vi "_testFileFlash.vi"(8 "speed":u32=4000, 9 "Path":path, 11 "implement":enum16{"Burning", "Erase"}(ring)) -> (10 "cmdStr out":string)   [LabVIEW 2020, in "LvJLinkARM.lvlib"]
uses:
  LvJLinkARM.lvlib
panel:
  out "return 5":i32
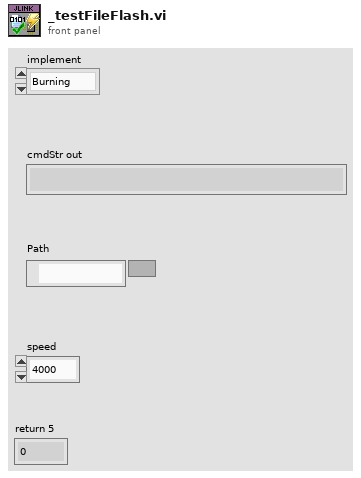
[diagram p1: front panel]
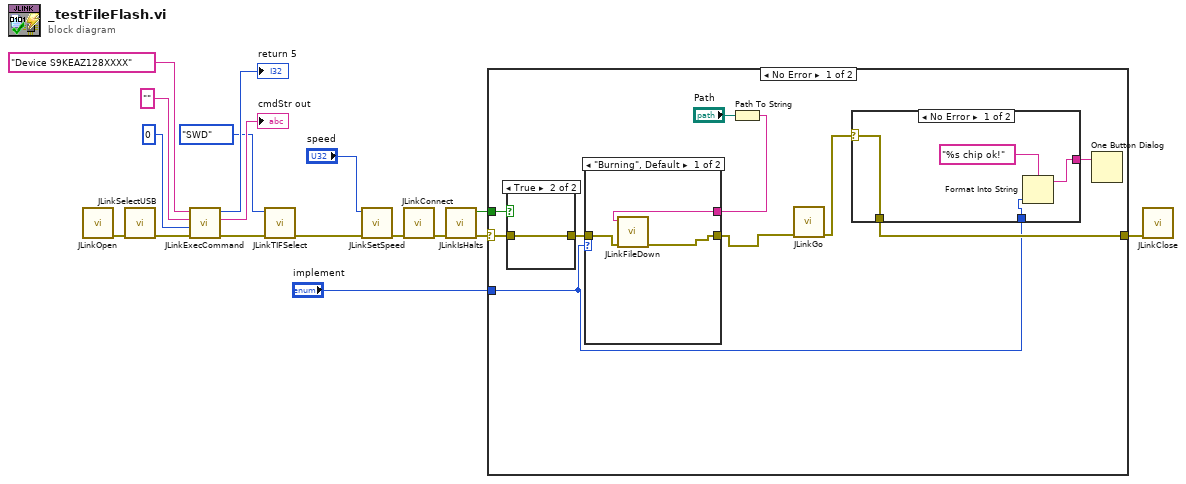
[diagram p0: block diagram]
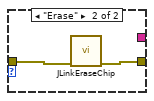
[diagram p2: hidden frame]
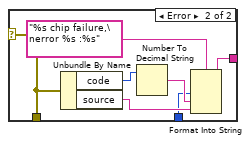
[diagram p3: hidden frame]
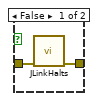
[diagram p4: hidden frame]
diagram:
  n1 = call "JLinkOpen.vi"() -> ("error out"=w7:errorcluster)  [unwired: 11 in]
  n2 = call "JLinkSelectUSB.vi"("error in (no error)"=w7) -> ("error out"=w8:errorcluster)  [unwired: 10 in]
  n3 = call "JLinkExecCommand.vi"("error in (no error)"=w8, "BufferSize"=0, "sError"="", "cmdStr"="Device S9KEAZ128XXXX") -> ("error out"=w11:errorcluster, "cmdStr out"=→"cmdStr out":string, "return"=→"return 5":i32)  [unwired: 5 in]
  n4 = call "JLinkTIFSelect.vi"("error in (no error)"=w11, "interface"=enum16{"JTAG", "SWD"}."SWD") -> ("error out"=w9:errorcluster)  [unwired: 9 in]
  n5 = call "JLinkSetSpeed.vi"("error in (no error)"=w9, "speed"="speed") -> ("error out"=w10:errorcluster)  [unwired: 9 in]
  n6 = call "JLinkConnect.vi"("error in (no error)"=w10) -> ("error out"=w5:errorcluster)  [unwired: 10 in]
  n7 = call "JLinkIsHalts.vi"("error in (no error)"=w5) -> ("error out"=w4:errorcluster, "inHalts？"=w3:bool)  [unwired: 9 in]
  n8 = case shown="No Error" w4 {
    selector: w4 -> [w26 w47]
    tunnel: w3 -> [w27 _]
    tunnel: [w23 w47] -> w2
    tunnel: "implement" -> [w18 _]
    frame No Error {
      n9 = case shown="True" w27 {
        tunnel: w26 -> [w45 w46]
        tunnel: [w44 w46] -> w25
        frame False {
          n10 = call "JLinkHalts.vi"("error in (no error)"=w45) -> ("error out"=w44:errorcluster)  [unwired: 9 in, 1 out]
        }
        frame True {
        }
      }
      n11 = Path To String(path="Path") -> (string=w21:string)
      n12 = case shown="\"Burning\", Default" w18 {
        tunnel: w25 -> [w29 w32]
        tunnel: [w28 w31] -> w20
        tunnel: w21 -> [w30 _]
        frame "Burning", Default {
          n13 = call "JLinkFileDown.vi"("error in (no error)"=w29, "sFileName"=w30) -> ("error out"=w28:errorcluster)  [unwired: 9 in]
        }
        frame "Erase" {
          n14 = call "JLinkEraseChip.vi"("error in (no error)"=w32) -> ("error out"=w31:errorcluster)  [unwired: 10 in]
        }
      }
      n15 = call "JLinkGo.vi"("error in (no error)"=w20) -> ("error out"=w19:errorcluster)  [unwired: 10 in]
      n16 = case shown="No Error" w19 {
        selector: w19 -> [w36 w43]
        tunnel: [w36 w43] -> w23
        tunnel: [w33 w42] -> w22
        tunnel: w18 -> [w35 w37]
        frame No Error {
          n17 = Format Into String(format string="%s chip ok!" ("message"), w35) -> (resulting string=w33:string)  [unwired: 2 in, 1 out]
        }
        frame Error {
          n18 = Unbundle By Name(w43) -> ("code"=w40:i32, "source"=w38:string)
          n19 = Number To Decimal String(number=w40) -> (decimal integer string=w39:string)  [unwired: 1 in]
          n20 = Format Into String(format string="%s chip failure,\nerror %s :%s", w37, w39, w38) -> (resulting string=w42:string)  [unwired: 2 in, 1 out]
        }
      }
      n21 = One Button Dialog(message=w22) -> ()  [unwired: 1 in, 1 out]
    }
    frame Error {
    }
  }
  n22 = call "JLinkClose.vi"("error in (no error)"=w2) -> ()  [unwired: 10 in, 1 out]
